vi "DHE_ReleaseHardSemaphore.vi"(8 "error in (no error)":errorcluster, 10 "release?":bool) -> (0 "error out":errorcluster)   [LabVIEW 2016]
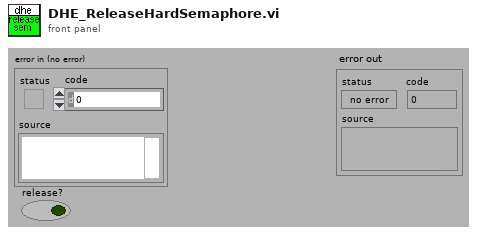
[diagram p1: front panel]
types:
  T1 = typedef "Semaphore RefNum" = refnum<k1>
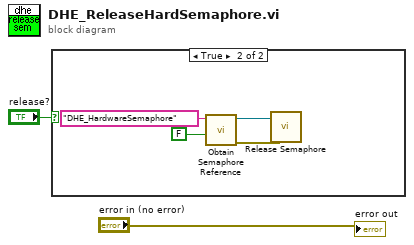
[diagram p0: block diagram]
diagram:
  n1 = case shown="True" "release?" {
    frame False {
    }
    frame True {
      n2 = call <vilib>:"Obtain Semaphore Reference.vi"("create if not found (T)"=FALSE, "name (unnamed)"="DHE_HardwareSemaphore") -> ("error out"=w3:errorcluster, "semaphore"=w4:T1)  [unwired: 2 in, 2 out]
      n3 = call <vilib>:"Release Semaphore.vi"("error in (no error)"=w3, "semaphore"=w4) -> ()  [unwired: 6 out]
    }
  }
  "error out" <- "error in (no error)"
